vi "Test Make Pairs two vlas.vi"(11 "Test Case In":refnum<class "Make Pairs Test.lvclass">) -> (0 "error out":errorcluster, 3 "Test Case Out":refnum<class "Make Pairs Test.lvclass">)   [LabVIEW 2020, in "Make Pairs Test.lvclass"]
uses:
  Make Pairs Test.lvclass
  C:/Program Files (x86)/National Instruments/LabVIEW 2020/vi.lib/Astemes/LUnit/Test Case.lvclass
  <vilib>/Astemes/LUnit/Test Case.lvclass/Test Case.ctl
  821d80fb-aeb4-4a7e-bf53-c941151ef697.vi
  4993e8ee-a06a-463a-9684-69129f64d5ce.vi
  <vilib>/Astemes/LUnit/Append Pass Result.vi
  <vilib>/Astemes/LUnit/Append Fail Result.vi
  <vilib>/Astemes/LUnit/Describe Comparison.vi
  4993e8ee-a06a-463a-9684-69129f64d5ce.vi/9c5d11cd-9439-4240-a1ee-d9baace9c924.vi
  <vilib>/Astemes/LUnit/Run In UI.vi
  <vilib>/Utility/error.llb/Clear Errors.vi
  <vilib>/Astemes/LUnit/Describe Variant.vi
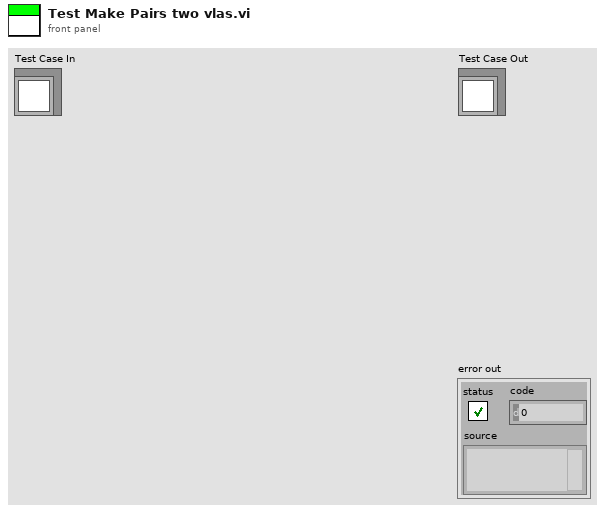
[diagram p1: front panel]
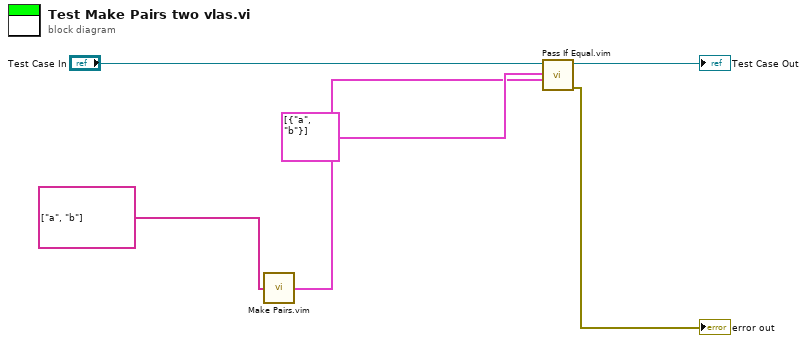
[diagram p0: block diagram]
diagram:
  n1 = call "Make Pairs.vim"("Array"=string[] ["a", "b"]) -> ("Pairs"=w1:cluster{string, string}[])
  n2 = call "Pass If Equal.vim"("Actual"=w1, "Expected"=cluster{string, string}[] [{"a", "b"}] ("Pairs"), "LUnit Test Case In"="Test Case In") -> ("error out"=→"error out":errorcluster, "LUnit Test Case Out"=→"Test Case Out":refnum<class "Make Pairs Test.lvclass">)  [unwired: 7 in]
